vi "Obtain.vi"(8 "Error In":errorcluster, 9 "Auto-reset on time elapsed (False)":bool, 10 "Time Goal (s)":dbl=1.0) -> (0 "Error Out":errorcluster, 3 "Timer Handle":T1)   [LabVIEW 2016, in "Timer Session.lvclass"]
doc: "This method creates a new timer that can be used for measuring time in your application.\n\nYou can use the reference given at the output or it's name to interact with it.\n\nBy default the timer is PAUSED. This means you have to call Enable Disable method to make it run."
uses:
  Timer Session.lvclass
  Typedefs/Session Handle.ctl
  Timer Session.lvclass/Timer Session.ctl
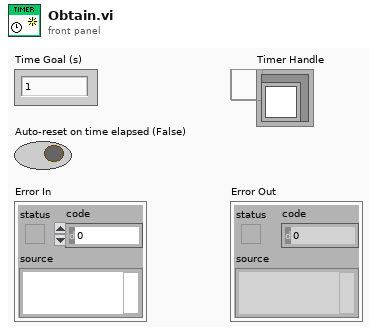
[diagram p1: front panel]
types:
  T1 = typedef "Timer Session.lvclass/Session Handle.ctl" = refnum<data-value>
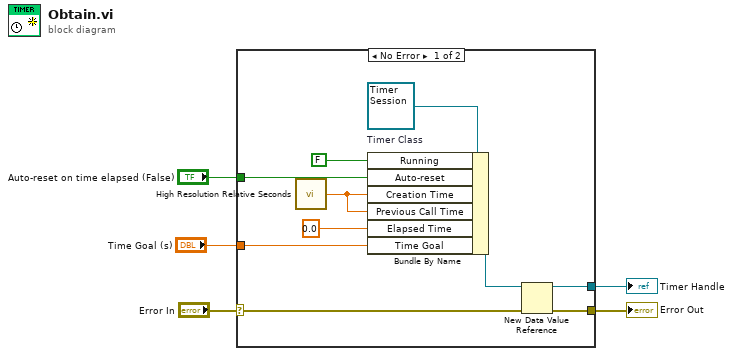
[diagram p0: block diagram]
diagram:
  n1 = case shown="No Error" "Error In" {
    selector: "Error In" -> [w8 w16]
    tunnel: [w6 w16] -> w4
    tunnel: [w7 _] -> w2
    tunnel: "Auto-reset on time elapsed (False)" -> [w15 _]
    tunnel: "Time Goal (s)" -> [w11 _]
    frame No Error {
      w14 = refnum<class "Timer Session.lvclass"> refnum  # Timer Class
      n2 = call <vilib>:"High Resolution Relative Seconds.vi"() -> ("relative seconds"=w13:dbl)
      n3 = Bundle By Name(cluster=w14, "Running"=FALSE, "Auto-reset"=w15, "Creation Time"=w13, "Previous Call Time"=w13, "Elapsed Time"=0.0 ("Start Time (ms)"), "Time Goal"=w11) -> (w9:refnum<class "Timer Session.lvclass">)
      n4 = New Data Value Reference(data value=w9, error in=w8) -> (data value reference=w7:refnum<data-value>, error out=w6:errorcluster)
    }
    frame Error {
    }
  }
  "Error Out" <- w4
  "Timer Handle" <- w2
